vi "Connect.vi"(8 "error in (no error)":errorcluster, 10 "Data Source":string, 11 "DatabaseBaseClass in":refnum<class "DatabaseBaseClass.lvclass">) -> (0 "error out":errorcluster, 3 "DatabaseBaseClass out":refnum<class "DatabaseBaseClass.lvclass">)   [LabVIEW 2018, in "Database.lvlib" / "DatabaseBaseClass.lvclass"]
uses:
  DatabaseBaseClass.lvclass
  DatabaseBaseClass.lvclass/DatabaseBaseClass.ctl
  <vilib>/addons/database/Connection.llb/DB Tools Open Connec (String).vi
  <vilib>/addons/database/NI_Database_API.lvlib
  Database.lvlib
panel:
  in  "btnStop":bool
  # "Connecting to Database..."
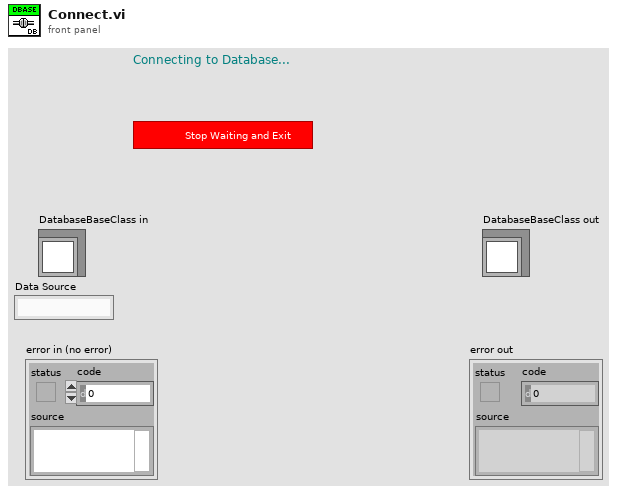
[diagram p1: front panel]
types:
  T1 = typedef "NI_Database_API.lvlib/Conn ObjectReference.ctl" = refnum<k1>
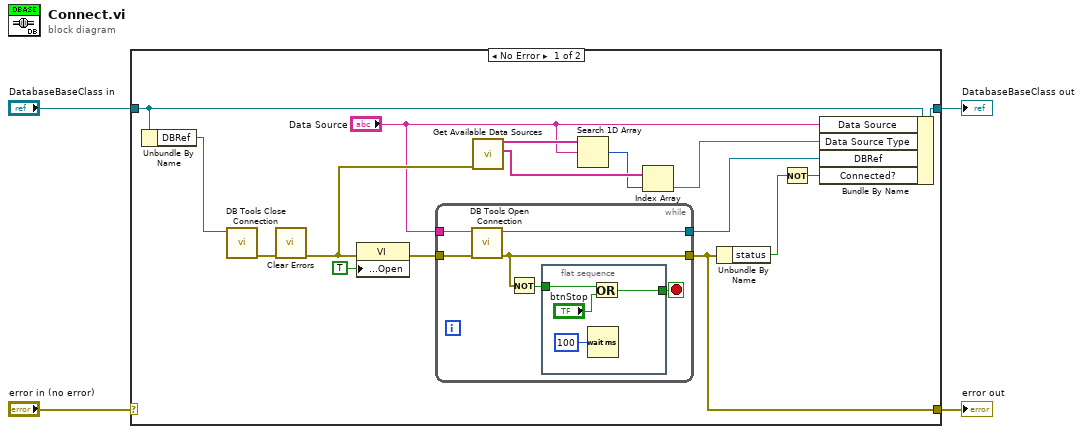
[diagram p0: block diagram]
diagram:
  n1 = case shown="No Error" "error in (no error)" {
    selector: "error in (no error)" -> [_ w32]
    tunnel: [w13 w32] -> w3
    tunnel: [w15 w31] -> w1
    tunnel: "DatabaseBaseClass in" -> [w17 w31]
    frame No Error {
      n2 = Unbundle By Name(w17) -> ("DBRef"=w16:T1)
      n3 = call <vilib>:"DB Tools Close Connection.vi"("connection reference"=w16) -> ("error out"=w18:errorcluster)  [unwired: 6 in]
      n4 = call <vilib>:"Clear Errors.vi"("error in (no error)"=w18) -> ("error out"=w10:errorcluster)  [unwired: 5 in, 1 out]
      n5 = property class="VI"(error in=w10, "Front Panel.Open"=TRUE ("Front Panel Window:Open")) -> (error out=w19:errorcluster)  [unwired: 1 in, 1 out]
      n6 = while {
        tunnel: "Data Source" -> [w26]
        tunnel: [w24] -> w14
        tunnel: w19 -> [w25]
        tunnel: [w23] -> w13
        stop <- w21 stop-if-true
        n7 = call-poly <vilib>:"DB Tools Open Connection.vi"("error in (no error)"=w25, "connection information"=w26) -> ("error out"=w23:errorcluster, "connection reference"=w24:T1)  [unwired: 6 in]
        n8 = Not(x=w23) -> (.not. x?=w22:bool)
        n9 = flat-sequence {
          tunnel: w22 -> [w30]
          tunnel: [w29] -> w21
          frame #0 {
            n10 = Wait (ms)(milliseconds to wait=u32 100) -> ()  [unwired: 1 out]
            n11 = Or(x=w30, y="btnStop") -> (x .or. y?=w29:bool)
          }
        }
      }
      n12 = call "Get Available Data Sources.vi"("error in (no error)"=w10) -> ("Data Source Type"=w7:string[], "Data Sources"=w9:string[])  [unwired: 8 in, 1 out]
      n13 = Search 1D Array(1D array=w9, element="Data Source") -> (index of element=w6:i32)  [unwired: 1 in]
      n14 = Index Array(array=w7, index=w6) -> (element=w5:string)
      n15 = Unbundle By Name(w13) -> ("status"=w12:bool)
      n16 = Not(x=w12) -> (.not. x?=w11:bool)
      n17 = Bundle By Name(cluster=w17, "Data Source"="Data Source", "Data Source Type"=w5, "DBRef"=w14, "Connected?"=w11) -> (w15:refnum<class "DatabaseBaseClass.lvclass">)
    }
    frame Error {
    }
  }
  "error out" <- w3
  "DatabaseBaseClass out" <- w1
